vi "Start.vi"() -> ()   [LabVIEW 2018]
uses:
  <vilib>/lvdsc/NI_DSC.lvlib
  <vilib>/lvdsc/security/NI Security Programmatic Login (Name).vi
panel:
  in  "Open visualisation":bool
  in  "stop":bool
  out "element":string
  out "logged in":bool
  in  "OK Button":bool
  in  "PASS":string
  in  "LOGIN":string
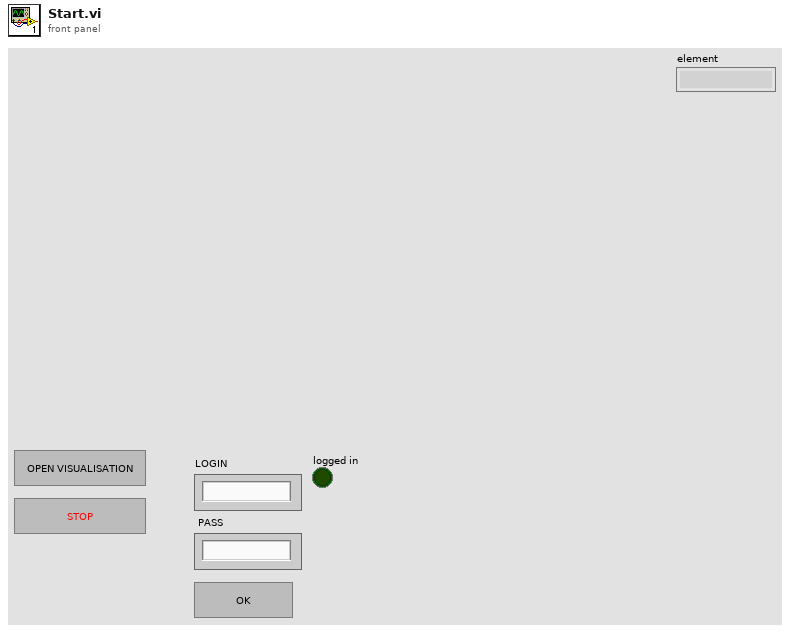
[diagram p1: front panel]
types:
  T1 = cluster{"status":bool, "code":bool, "source":bool}
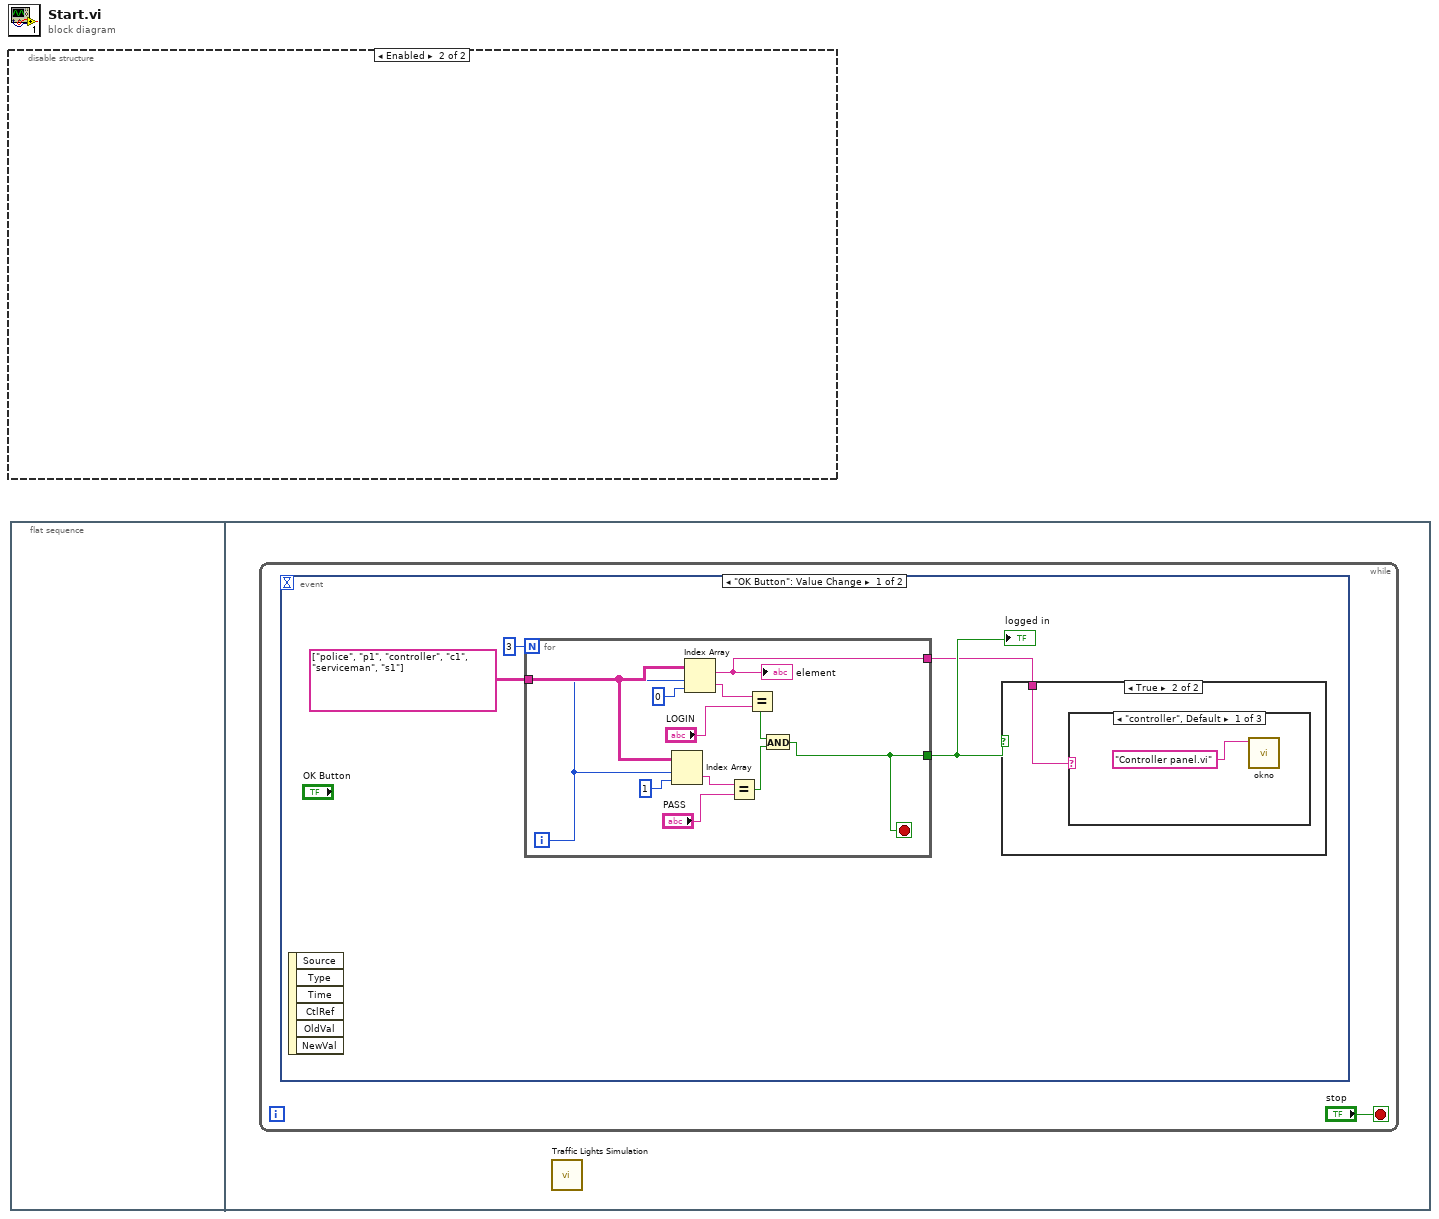
[diagram p0: block diagram]
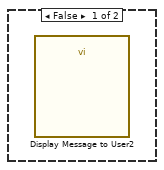
[diagram p2: hidden frame]
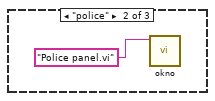
[diagram p3: hidden frame]
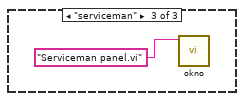
[diagram p4: hidden frame]
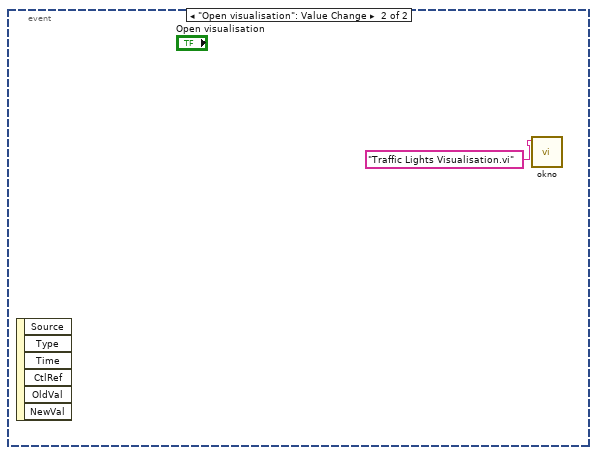
[diagram p5: hidden frame]
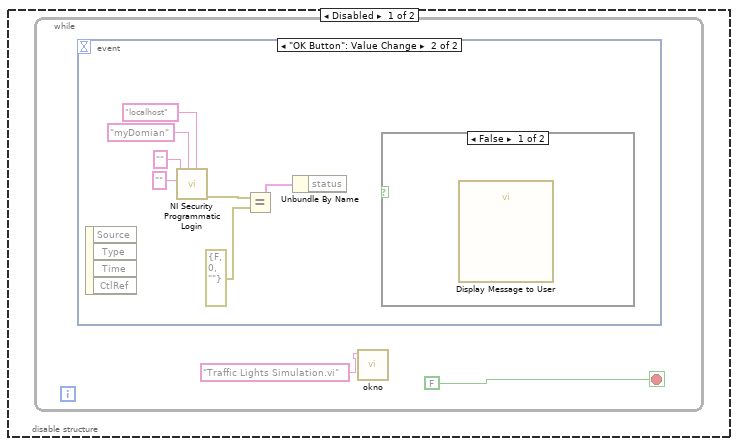
[diagram p6: hidden frame]
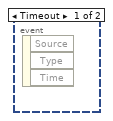
[diagram p7: hidden frame]
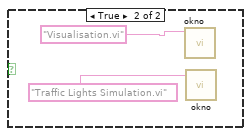
[diagram p8: hidden frame]
diagram:
  n1 = disable-structure shown="Enabled" {
    frame Disabled {
      n2 = while {
        stop <- FALSE stop-if-true
        n3 = event shown="[1] \"OK Button\": Value Change" {
          selector: _ -> [_ _]
          dyn-events: _ -> [_ _]
          timeout: _ -> [_ _]
          event Timeout {
            n4 = event-data() -> ()  [unwired: 1 in, 3 out]
          }
          event "OK Button": Value Change {
            n5 = event-data() -> ()  [unwired: 1 in, 4 out]
            n6 = call-poly <vilib>:"NI Security Programmatic Login.vi"("domain machine"="localhost", "domain name"="myDomian", "password"="", "user name"="") -> ("error out"=w7:errorcluster)  [unwired: 5 in, 2 out]
            n7 = Equal?(x=w7, y=errorcluster {"status"=FALSE, "code"=0, "source"=""}) -> (x = y?=w5:T1)
            n8 = Unbundle By Name(w5) -> ()  [unwired: 1 out]
            n9 = case shown="False" {
              selector: _ -> [_ _]
              frame False {
                n10 = call "Display Message to User"() -> ()  [unwired: 10 in, 2 out]
              }
              frame True {
                n11 = call "okno.vi"("name or relative path"="Visualisation.vi") -> ()  [unwired: 11 in]
                n12 = call "okno.vi"("name or relative path"="Traffic Lights Simulation.vi") -> ()  [unwired: 11 in]
              }
            }
          }
        }
        n13 = call "okno.vi"("name or relative path"="Traffic Lights Simulation.vi") -> ()  [unwired: 11 in]
      }
    }
    frame Enabled {
    }
  }
  n14 = flat-sequence {
    frame #0 {
    }
    frame #1 {
      n15 = while {
        stop <- "stop" stop-if-true
        n16 = event shown="[0] \"OK Button\": Value Change" {
          selector: _ -> [_ _]
          dyn-events: _ -> [_ _]
          timeout: _ -> [_ _]
          event "OK Button": Value Change {
            n17 = event-data() -> ()  [unwired: 1 in, 6 out]
            n18 = for {
              N: 3 -> [_]
              tunnel: [w21] -> w14
              tunnel: string[][] [["police", "p1"], ["controller", "c1"], ["serviceman", "s1"]] -> [w24]
              tunnel: [w22] -> w13
              i -> [w23]
              stop <- w21 stop-if-true
              n19 = Index Array(array=w24, index (row)=w23, index (col)=1 ("disabled index (col)")) -> (element=w25:string)
              n20 = Index Array(array=w24, index (row)=w23, index (col)=0 ("disabled index (col)")) -> (element=w22:string)
              "element" <- w22
              n21 = Equal?(x=w25, y="PASS") -> (x = y?=w28:bool)
              n22 = Equal?(x=w22, y="LOGIN") -> (x = y?=w29:bool)
              n23 = And(x=w29, y=w28) -> (x .and. y?=w21:bool)
            }
            "logged in" <- w14
            n24 = case shown="True" w14 {
              tunnel: w13 -> [_ w17]
              frame False {
                n25 = call "Display Message to User2"() -> ()  [unwired: 10 in, 2 out]
              }
              frame True {
                n26 = case shown="\"controller\", Default" w17 {
                  frame "controller", Default {
                    n27 = call "okno.vi"("name or relative path"="Controller panel.vi") -> ()  [unwired: 11 in]
                  }
                  frame "police" {
                    n28 = call "okno.vi"("name or relative path"="Police panel.vi") -> ()  [unwired: 11 in]
                  }
                  frame "serviceman" {
                    n29 = call "okno.vi"("name or relative path"="Serviceman panel.vi") -> ()  [unwired: 11 in]
                  }
                }
              }
            }
          }
          event "Open visualisation": Value Change {
            n30 = event-data() -> ()  [unwired: 1 in, 6 out]
            n31 = call "okno.vi"("name or relative path"="Traffic Lights Visualisation.vi") -> ()  [unwired: 11 in]
          }
        }
      }
      n32 = call "Traffic Lights Simulation.vi"() -> ()  [unwired: 12 in]
    }
  }
